vi "ChangeLane.vi"(6 "Lane":i32, 7 "offset":dbl, 8 "Pose (X, Y, Theta)":dbl[](array[numeric]), 9 "Switch":cluster{"SwitchRight":bool, "SwitchLeft":bool}, 10 "Trajectory In":cluster{"X":dbl[], "Y":dbl[], "Theta":dbl[]}, 11 "Lanes":T1) -> (3 "Trajectory out":cluster{"X":dbl[], "Y":dbl[], "Theta":dbl[]})   [LabVIEW 2013]
uses:
  <vilib>/imath/engines/lvmath2/RunTimeEngine/ErrorHandling/NIMS_Finalize Error.vi
  <vilib>/imath/engines/lvmath2/RunTimeEngine/Managers/WorkSpace/UID Generator.vi
  <vilib>/imath/engines/lvmath2/RunTimeEngine/Managers/SymbolTable/Clear UID.vi
  <vilib>/imath/engines/lvmath2/RunTimeEngine/NodeEndStatement/NIMS_NodeEndStatement_Output.vi
  <instcachedir>/0/NIMS_NodeEndStatement_Output_53EC0D466D134D7ABD903AC30B43404B.lvgen/NIMS_NodeEndStatement_Output_53EC0D466D134D7ABD903AC30B43404B_005.vi
  <vilib>/imath/engines/lvmath2/RunTimeEngine/RunTimeType/NIMS_RunTimeType_From StrictType (excl LVString).vi
  <instcachedir>/0/NIMS_RunTimeType_From StrictType (excl LVString)_4DEE718D6EB74582AA20236969C084FC.lvgen/NIMS_RunTimeType_From StrictType (excl LVString)_4DEE718D6EB74582AA20236969C084FC_000.vi
  <vilib>/imath/engines/lvmath2/RunTimeEngine/LocalVariableDefStatement/MC_LocalVariableDefStatement_Display.vi
  <vilib>/imath/engines/lvmath2/RunTimeEngine/VariableToken/NIMS_VariableToken_CondDefined.vi
  <instcachedir>/0/NIMS_VariableToken_CondDefined_9DC5CEC47F8146B087FA2781C705B229.lvgen/NIMS_VariableToken_CondDefined_9DC5CEC47F8146B087FA2781C705B229_001.vi
  <vilib>/imath/engines/lvmath2/RunTimeEngine/IndexRead/NIMS M($,S).vi
  <instcachedir>/0/NIMS M($,S)_3E5749BBB62E49528D4765A77F1F6D98.lvgen/NIMS M($,S)_3E5749BBB62E49528D4765A77F1F6D98_000.vi
  <vilib>/imath/engines/lvmath2/RunTimeEngine/ArithmeticOperatorToken/NIMS_ArithmeticOperator_plus.vi
  <instcachedir>/0/NIMS_ArithmeticOperator_plus_8A46DAFC24D445C9B2C97B626139369E.lvgen/NIMS_ArithmeticOperator_plus_8A46DAFC24D445C9B2C97B626139369E_004.vi
  <vilib>/imath/engines/lvmath2/RunTimeEngine/ErrorHandling/NIMS_Create Error From Enums.vi
  <vilib>/imath/engines/lvmath2/RunTimeEngine/IndexRead/NIMS V(S).vi
  <instcachedir>/0/NIMS V(S)_0488751826AF41519A22953C041130DC.lvgen/NIMS V(S)_0488751826AF41519A22953C041130DC_000.vi
  <vilib>/imath/engines/lvmath2/RunTimeEngine/BuiltInFunctions/min/1 input/NIMS_min(CV).vi
  <instcachedir>/0/NIMS_min(CV)_46E60952406B4159AB512BDF500C959F.lvgen/NIMS_min(CV)_46E60952406B4159AB512BDF500C959F_000.vi
  <vilib>/imath/engines/lvmath2/RunTimeEngine/BuiltInFunctions/length/NIMS_length(GV).vi
  <instcachedir>/0/NIMS_length(GV)_08A3D13377FD4E4B96F5795FBF3698FA.lvgen/NIMS_length(GV)_08A3D13377FD4E4B96F5795FBF3698FA_000.vi
  <vilib>/imath/engines/lvmath2/RunTimeEngine/Managers/SymbolTable/NIMS_WorkSpace.lvlib
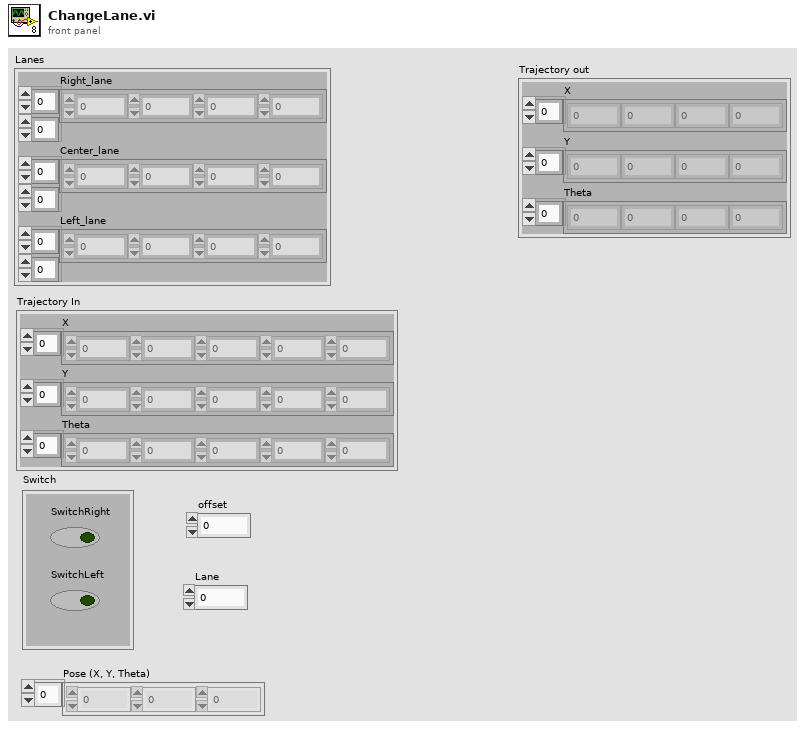
[diagram p1: front panel]
types:
  T1 = cluster{"Right_lane":dbl[][], "Center_lane":dbl[][], "Left_lane":dbl[][]}
  T2 = cluster{"Current Position":dbl[], "Current lane":dbl, "SwitchRight":bool, "SwitchLeft":bool}
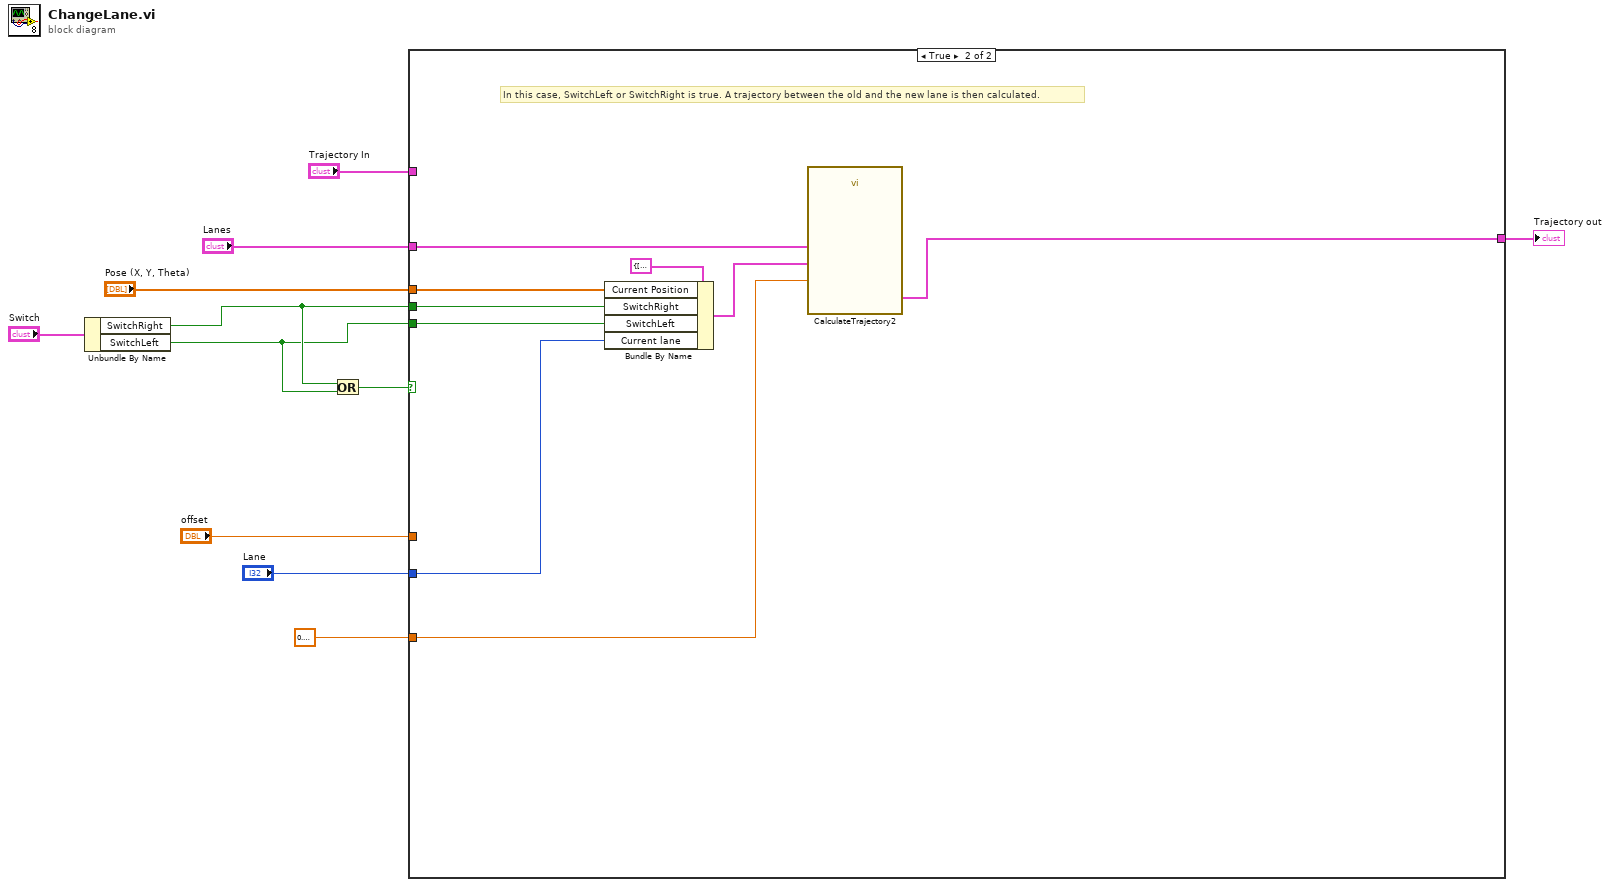
[diagram p0: block diagram]
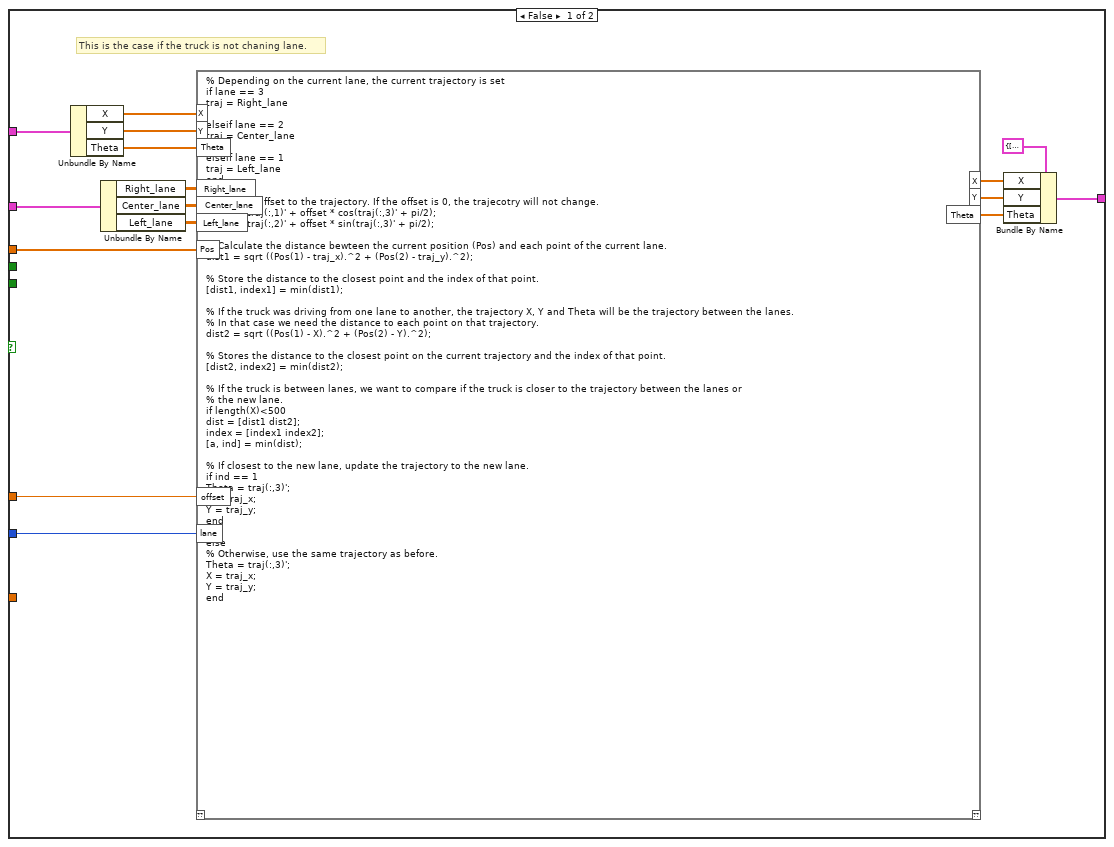
[diagram p2: hidden frame]
diagram:
  n1 = Unbundle By Name("Switch") -> ("SwitchRight"=w3:bool, "SwitchLeft"=w2:bool)
  n2 = Or(x=w3, y=w2) -> (x .or. y?=w11:bool)
  n3 = case shown="True" w11 {
    tunnel: [w23 w472] -> w10
    tunnel: "Lanes" -> [w14 w473]
    tunnel: "Pose (X, Y, Theta)" -> [w18 w480]
    tunnel: "Lane" -> [w12 w476]
    tunnel: w2 -> [_ w477]
    tunnel: w3 -> [_ w478]
    tunnel: "Trajectory In" -> [w22 _]
    tunnel: 0.7999999999999996 ("LaneChangeDistance") -> [_ w475]
    tunnel: "offset" -> [w13 _]
    frame False {
      # "This is the case if the truck is not chaning lane."
      n4 = Unbundle By Name(w22) -> ("X"=w21:dbl[], "Y"=w20:dbl[], "Theta"=w19:dbl[])
      n5 = Unbundle By Name(w14) -> ("Right_lane"=w27:dbl[][], "Center_lane"=w25:dbl[][], "Left_lane"=w26:dbl[][])
      n6 = mathscript code="% Depending on the current lane, the current trajectory is set\nif lane == 3\ntraj = Right_lane\n\nelseif lane == 2\ntraj = Center_lane\n\nelseif lane == 1\ntraj = Left_lane\nend\n\n% Add the offset to the trajectory. If the offset is 0, the trajecotry will not change.\ntraj_x = traj(:,1)' + offset * cos(traj(:,3)' + pi/2);\ntraj_y = traj(:,2)' + offset * sin(traj(:,3)' + pi/2);\n\n% Calculate the distance bewteen the current position (Pos) and each point of the current lane.\ndist1 = sqrt ((Pos(1) - traj_x).^2 + (Pos(2) - traj_y).^2);\n\n% Store the distance to the closest point and the index of that point.\n[dist1, index1] = min(dist1);\n\n% If the truck was driving from one lane to another, the trajectory X, Y and Theta will be the trajectory between the lanes.\n% In that case we need the distance to each point on that trajectory.\ndist2 = sqrt ((Pos(1) - X).^2 + (Pos(2) - Y).^2);\n\n% Stores the distance to the closest point on the current trajectory and the index of that point.\n[dist2, index2] = min(dist2);\n\n% If the truck is between lanes, we want to compare if the truck is closer to the trajectory between the lanes or\n% the new lane. \nif length(X)<500\ndist = [dist1 dist2];\nindex = [index1 index2];\n[a, ind] = min(dist);\n\n% If closest to the new lane, update the trajectory to the new lane.\nif ind == 1\nTheta = traj(:,3)';\nX = traj_x;\nY = traj_y;\nend\n\nelse\n% Otherwise, use the same trajectory as before.\nTheta = traj(:,3)';\nX = traj_x;\nY = traj_y;\nend"("lane"=w12, "Right_lane"=w27, "Center_lane"=w25, "Left_lane"=w26, "X"=w21, "Y"=w20, "Theta"=w19, "Pos"=w18, "offset"=w13) -> ("X"=w17:dbl[], "Y"=w16:dbl[], "Theta"=w15:dbl[])  [unwired: 1 in, 1 out]
      n7 = Bundle By Name(cluster=cluster{"X":dbl[], "Y":dbl[], "Theta":dbl[]} {"X"=[], "Y"=[], "Theta"=[]} ("Cluster"), "X"=w17, "Y"=w16, "Theta"=w15) -> (w23:cluster{"X":dbl[], "Y":dbl[], "Theta":dbl[]})
    }
    frame True {
      # "In this case, SwitchLeft or SwitchRight is true. A trajectory between the old and the new lane is then calculated."
      n8 = Bundle By Name(cluster=T2 {"Current Position"=[], "Current lane"=1.0, "SwitchRight"=FALSE, "SwitchLeft"=FALSE} ("Inputs"), "Current Position"=w480, "SwitchRight"=w478, "SwitchLeft"=w477, "Current lane"=w476) -> (w474:T2)
      n9 = call "CalculateTrajectory2.vi"("ChangingDistance"=w475, "Inputs"=w474, "Lanes"=w473) -> ("Trajectory"=w472:cluster{"X":dbl[], "Y":dbl[], "Theta":dbl[]})  [unwired: 8 in]
    }
  }
  "Trajectory out" <- w10
